vi "Check for Reboot Loop.vi"(8 "error in (no error)":errorcluster) -> (0 "error out":errorcluster, 2 "Start in Safe Mode?":bool)   [LabVIEW 2015]
uses:
  Globals/Global - Configuration Options.vi
  <vilib>/Utility/file.llb/Read Delimited Spreadsheet (string).vi
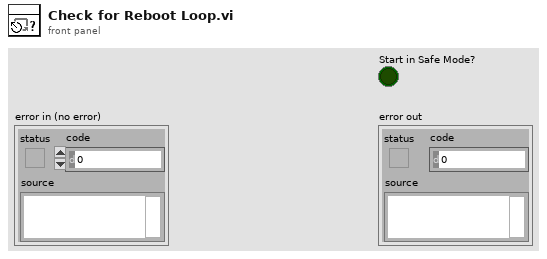
[diagram p1: front panel]
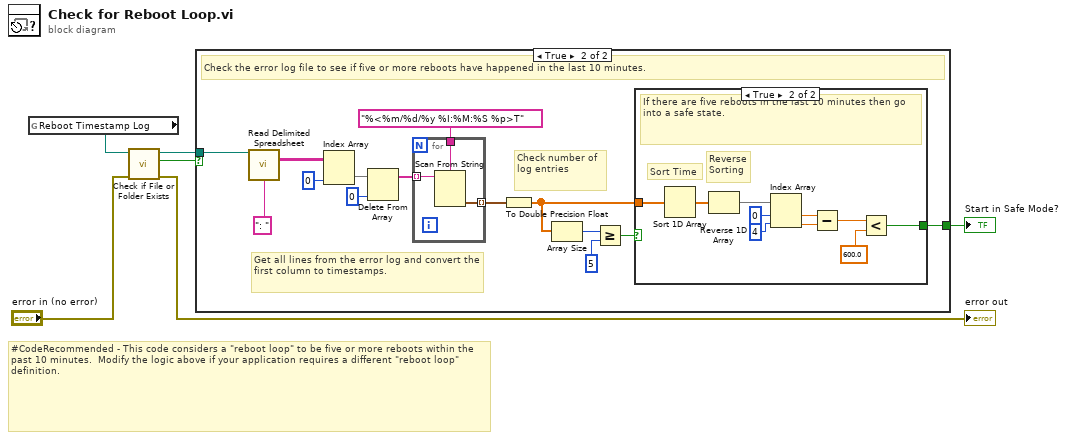
[diagram p0: block diagram]
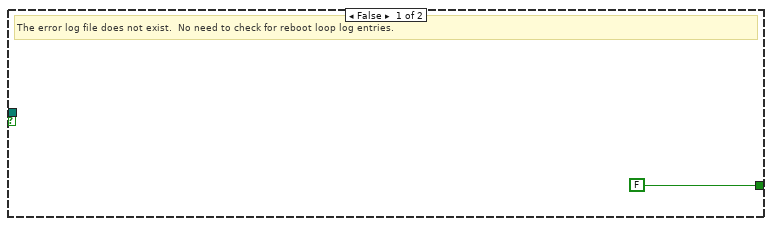
[diagram p2: hidden frame]
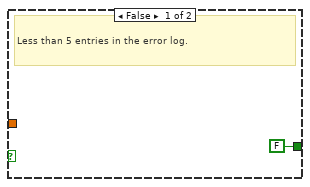
[diagram p3: hidden frame]
diagram:
  # "#CodeRecommended - This code considers a \"reboot loop\" to be five or more reboots within the past 10 minutes.  Modify the logic above if your application requires a different \"reboot loop\" definition."
  n1 = global read "Global - Configuration Options.vi" "Reboot Timestamp Log"() -> (w1:path)
  n2 = call <vilib>:"Check if File or Folder Exists.vi"("error in (no error)"="error in (no error)", "path"=w1) -> ("error out"=→"error out":errorcluster, "file or folder exists?"=w4:bool, "dup path"=w3:path)  [unwired: 7 in]
  n3 = case shown="True" w4 {
    tunnel: w3 -> [_ w21]
    tunnel: [FALSE w17] -> w2
    frame False {
      # "The error log file does not exist.  No need to check for reboot loop log entries."
    }
    frame True {
      # "Check number of log entries"
      # "Get all lines from the error log and convert the first column to timestamps."
      # "Check the error log file to see if five or more reboots have happened in the last 10 minutes."
      n4 = call-poly <vilib>:"Read Delimited Spreadsheet.vi"("file path (dialog if empty)"=w21, "delimiter (\\t)"=": " ("delimiter (\\t)")) -> ("all rows"=w8:string[][])  [unwired: 8 in, 5 out]
      n5 = Index Array(array=w8, index (col)=0 ("disabled index (col)")) -> (element=w11:string[])  [unwired: 1 in]
      n6 = Delete From Array(array=w11, index=0) -> (array with subset deleted=w10:string[])  [unwired: 1 in, 1 out]
      n7 = for {
        tunnel: w10 -> [w35] mode=indexing
        tunnel: "%<%m/%d/%y %I:%M:%S %p>T" -> [w34]
        tunnel: [w33] -> w18 mode=indexing
        n8 = Scan From String(format string=w34, input string=w35) -> (output 1=w33:timestamp)  [unwired: 3 in, 3 out]
      }
      n9 = To Double Precision Float(number=w18) -> (double precision float=w16:dbl[])
      n10 = Array Size(array=w16) -> (size(s)=w15:i32)
      n11 = Greater Or Equal?(x=w15, y=5) -> (x >= y?=w13:bool)
      n12 = case shown="True" w13 {
        tunnel: [FALSE w24] -> w17
        tunnel: w16 -> [_ w23]
        frame False {
          # "Less than 5 entries in the error log."
        }
        frame True {
          # "Reverse\nSorting"
          # "Sort Time"
          # "If there are five reboots in the last 10 minutes then go into a safe state."
          n13 = Sort 1D Array(array=w23) -> (sorted array=w32:dbl[])
          n14 = Reverse 1D Array(array=w32) -> (reversed array=w31:dbl[])
          n15 = Index Array(array=w31, index #1=0 ("index"), index #2=4 ("index")) -> (element #1=w28:dbl, element #2=w27:dbl)
          n16 = Subtract(x=w28, y=w27) -> (x-y=w26:dbl)
          n17 = Less?(x=w26, y=600.0) -> (x < y?=w24:bool)
        }
      }
    }
  }
  "Start in Safe Mode?" <- w2
